vi "Handle Last Ack Core.vi"(4 "error in (no error)":errorcluster, 6 "Last Ack":refnum<class "Last Ack.lvclass">, 7 "PLC Sim Controller Actor in":refnum<class "PLC Sim Controller Actor.lvclass">) -> (0 "error out":errorcluster, 3 "PLC Sim Controller Actor out":refnum<class "PLC Sim Controller Actor.lvclass">)   [LabVIEW 2019, in "PLC Sim Controller Actor.lvlib" / "PLC Sim Controller Actor.lvclass"]
doc: "(<B>Filename</B>: Actor Framework.lvlib:Actor.lvclass:Handle Last Ack Core.vi)\n\nDefines how the caller actor responds to the Last Ack message from a nested actor. The Last Ack message is the final message a nested actor sends to its caller before it shuts down. The message contains information about the final state of the nested actor.\n\nBy default, this method does nothing except return any error the nested actor sent. A descendant class may override this method to define behavior."
uses:
  PLC Sim Controller Actor.lvclass
  <vilib>/ActorFramework/LastAck/Last Ack.lvclass
  PLC Sim Controller Actor.lvclass/PLC Sim Controller Actor.ctl
  <vilib>/ActorFramework/Actor/Actor.lvclass
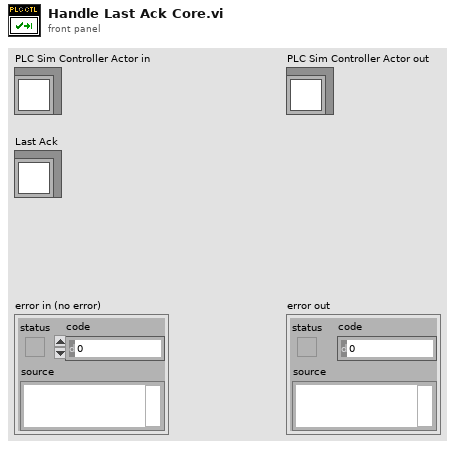
[diagram p1: front panel]
types:
  T1 = map{string, refnum<class "Message Enqueuer.lvclass">}
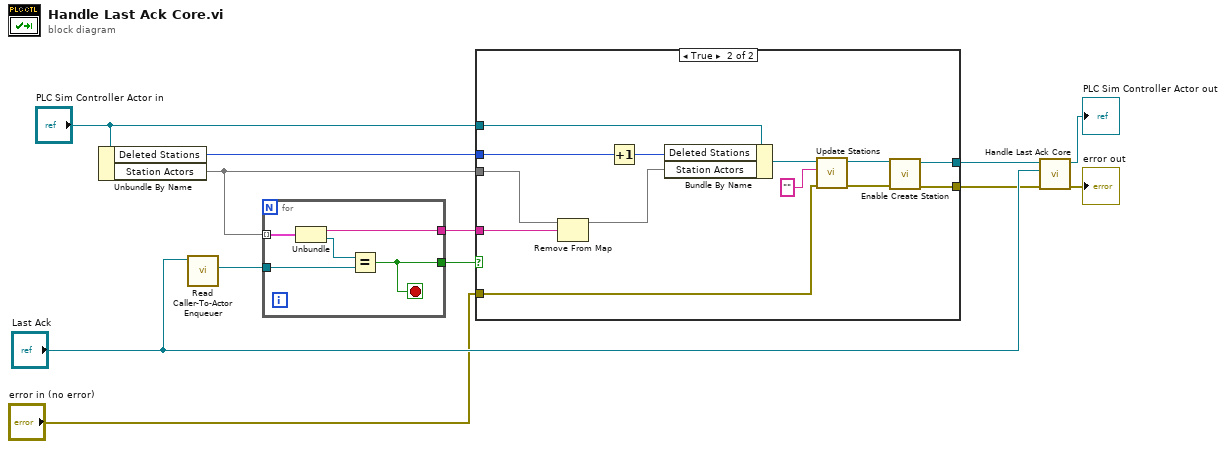
[diagram p0: block diagram]
diagram:
  n1 = Unbundle By Name("PLC Sim Controller Actor in") -> ("Deleted Stations"=w5:u32, "Station Actors"=w8:T1)
  n2 = call <vilib>:"Read Caller-To-Actor Enqueuer.vi"("Last Ack"="Last Ack") -> ("Caller-to-Actor Enqueuer"=w9:refnum<class "Message Enqueuer.lvclass">)  [unwired: 10 in]
  n3 = for {
    tunnel: w8 -> [w17] mode=indexing
    tunnel: w9 -> [w16]
    tunnel: [w14] -> w7
    tunnel: [w13] -> w6
    stop <- w14 stop-if-true
    n4 = Unbundle(w17) -> (w13:string, "Station Enqueuer"=w15:refnum<class "Message Enqueuer.lvclass">)
    n5 = Equal?(x=w15, y=w16) -> (x = y?=w14:bool)
  }
  n6 = case shown="True" w7 {
    tunnel: w8 -> [_ w30]
    tunnel: w6 -> [_ w20]
    tunnel: w5 -> [_ w29]
    tunnel: "PLC Sim Controller Actor in" -> [w19 w28]
    tunnel: "error in (no error)" -> [w18 w23]
    tunnel: [w18 w22] -> w2
    tunnel: [w19 w21] -> w1
    frame False {
    }
    frame True {
      n7 = Remove From Map(10:w20, 11:w30) -> (3:w31:T1)  [unwired: 2 out]
      n8 = Increment(x=w29) -> (x+1=w32:u32)
      n9 = Bundle By Name(cluster=w28, "Deleted Stations"=w32, "Station Actors"=w31) -> (w27:refnum<class "PLC Sim Controller Actor.lvclass">)
      n10 = call "Update Stations.vi"("error in (no error)"=w23, "Combo Value"="", "OPC Server in"=w27) -> ("error out"=w24:errorcluster, "OPC Server out"=w25:refnum<class "PLC Sim Controller Actor.lvclass">)  [unwired: 7 in]
      n11 = call "Enable Create Station.vi"("error in (no error)"=w24, "PLC Sim Controller Actor in"=w25) -> ("error out"=w22:errorcluster, "PLC Sim Controller Actor out"=w21:refnum<class "PLC Sim Controller Actor.lvclass">)  [unwired: 8 in]
    }
  }
  n12 = call-parent "Handle Last Ack Core.vi"("error in (no error)"=w2, "Last Ack"="Last Ack", "Actor in"=w1) -> ("error out"=→"error out":errorcluster, "Actor out"=→"PLC Sim Controller Actor out":refnum<class "PLC Sim Controller Actor.lvclass">)  [unwired: 3 in]
